vi "Get Methods (SubVI).vi"(8 "error in (no error)":errorcluster, 11 "VISA Refnum in":refnum<visa-resource-name>) -> (0 "error out":errorcluster, 1 "Array":string[](array[string]), 2 "Response":string, 3 "VISA Refnum out":refnum<visa-resource-name>)   [LabVIEW 2013]
panel:
  in  "Command":string="?"
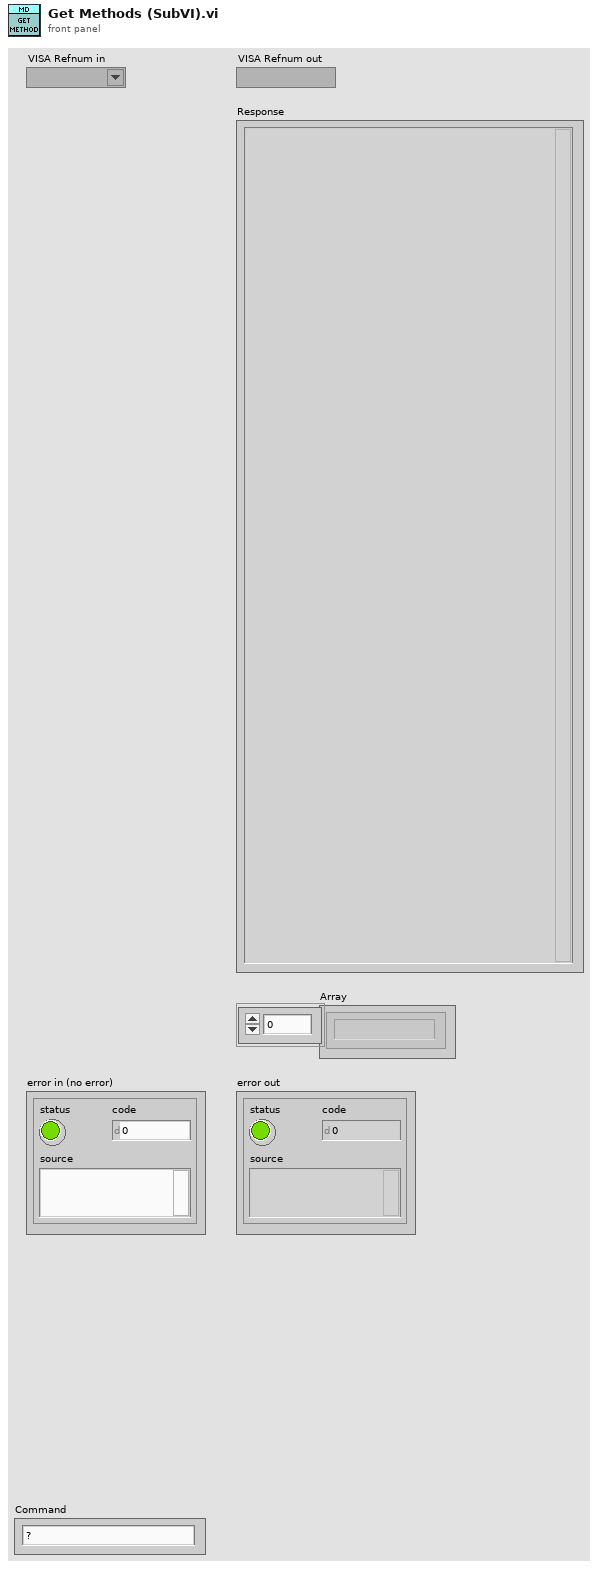
[diagram p1: front panel]
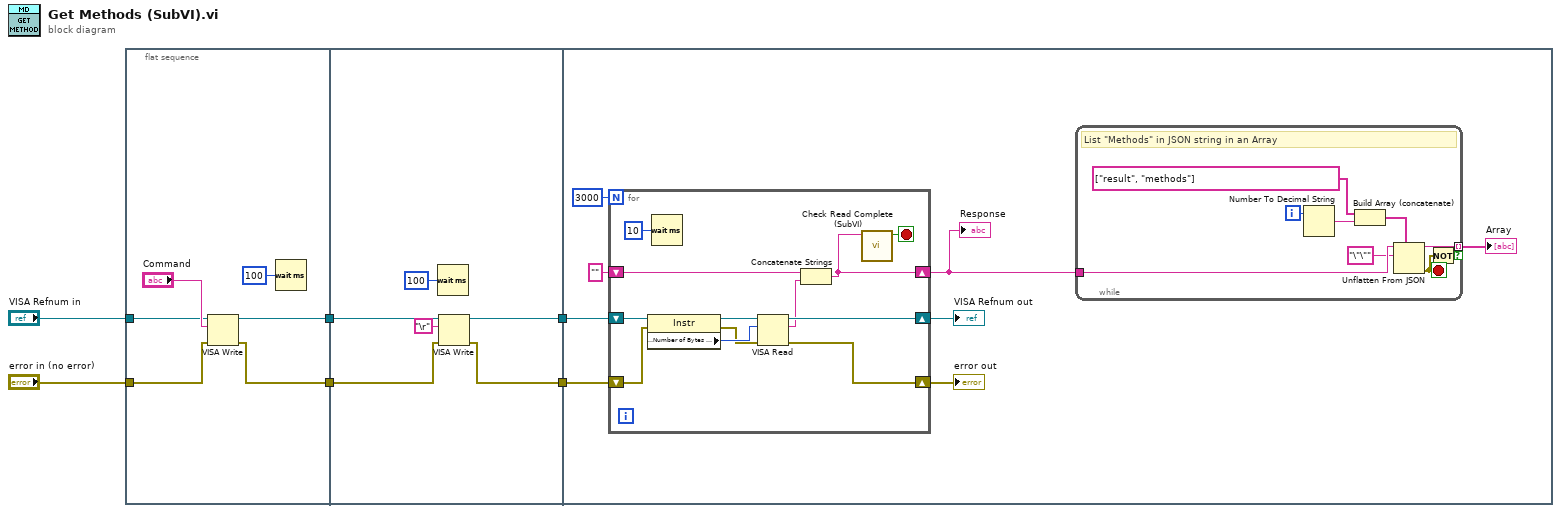
[diagram p0: block diagram]
diagram:
  n1 = flat-sequence {
    tunnel: "VISA Refnum in" -> [w10]
    tunnel: "error in (no error)" -> [w8]
    tunnel: [w7] -> w2
    tunnel: [w9] -> w1
    tunnel: [w13] -> w4
    tunnel: [w15] -> w3
    tunnel: w2 -> [w14]
    tunnel: w1 -> [w16]
    tunnel: w4 -> [w25]
    tunnel: w3 -> [w24]
    frame #0 {
      n2 = VISA Write(VISA resource name=w10, write buffer="Command", error in (no error)=w8) -> (VISA resource name out=w9:refnum<visa-resource-name>, error out=w7:errorcluster)  [unwired: 1 out]
      n3 = Wait (ms)(milliseconds to wait=u32 100) -> ()  [unwired: 1 out]
    }
    frame #1 {
      n4 = Wait (ms)(milliseconds to wait=u32 100) -> ()  [unwired: 1 out]
      n5 = VISA Write(VISA resource name=w16, write buffer="\r", error in (no error)=w14) -> (VISA resource name out=w15:refnum<visa-resource-name>, error out=w13:errorcluster)  [unwired: 1 out]
    }
    frame #2 {
      n6 = for {
        N: 3000 -> [_]
        shift-right: [w47] -> w22
        shift-left: w24 -> [w45]
        shift-right: [w46] -> w23
        shift-left: w25 -> [w39]
        shift-right: [w36] -> w19
        shift-left: "" -> [w41]
        stop <- w37 stop-if-true
        n7 = property class="Instr"(reference=w45, error in=w39) -> (reference out=w43:refnum<visa-resource-name>, error out=w38:errorcluster, "Serial Settings:Number of Bytes at Serial Port"=w42:u32)
        n8 = Wait (ms)(milliseconds to wait=u32 10) -> ()  [unwired: 1 out]
        n9 = VISA Read(VISA resource name=w43, byte count=w42, error in (no error)=w38) -> (VISA resource name out=w47:refnum<visa-resource-name>, read buffer=w44:string, error out=w46:errorcluster)  [unwired: 1 out]
        n10 = Concatenate Strings(w41, w44) -> (w36:string)
        n11 = call "Check Read Complete (SubVI).vi"("JSON String"=w36) -> ("Complete?"=w37:bool)  [unwired: 10 in]
      }
      "error out" <- w23
      "VISA Refnum out" <- w22
      "Response" <- w19
      n12 = while {
        tunnel: w19 -> [w35]
        tunnel: [w33] -> w26 mode=indexing if=w27
        i -> [w30]
        stop <- w28 stop-if-true
        # "List \"Methods\" in JSON string in an Array"
        n13 = Number To Decimal String(number=w30) -> (decimal integer string=w31:string)  [unwired: 1 in]
        n14 = Build Array (concatenate)(string[] ["result", "methods"], w31) -> (w32:string[])
        n15 = Unflatten From JSON(path=w32, JSON string=w35, type and defaults="\"\"" ("JSON string")) -> (value=w33:string, error out=w28:errorcluster)  [unwired: 4 in]
        n16 = Not(x=w28) -> (.not. x?=w27:bool)
      }
      "Array" <- w26
    }
  }
